vi "Log Error.vi"(8 "error in (no error)":errorcluster, 9 "error to log (no error)":errorcluster, 10 "Source Name":string, 11 "cRIO-CO2 in":refnum<class "cRIO-CO2.lvclass">) -> (0 "error out":errorcluster, 3 "cRIO-CO2 out":refnum<class "cRIO-CO2.lvclass">)   [LabVIEW 2015, in "cRIO-Carbondioxide.lvlib" / "cRIO-CO2.lvlib" / "cRIO-CO2.lvclass"]
uses:
  cRIO-CO2.lvclass
  <vilib>/Utility/error.llb/DialogType.ctl
  cRIO-CO2.lvclass/cRIO-CO2.ctl
  cRIO-CO2 Messages/Log Message Msg/Log Message Msg.lvclass/Log Message Msg.ctl
  <vilib>/ActorFramework/Message Enqueuer/Message Enqueuer.lvclass/Message Enqueuer.ctl
  <vilib>/ActorFramework/Message Enqueuer/Enqueue.vi
  <vilib>/ActorFramework/Message Priority Queue/Priority Enqueue.vi
  cRIO-CO2 Messages/Log Message Msg/Log Message Msg.lvclass
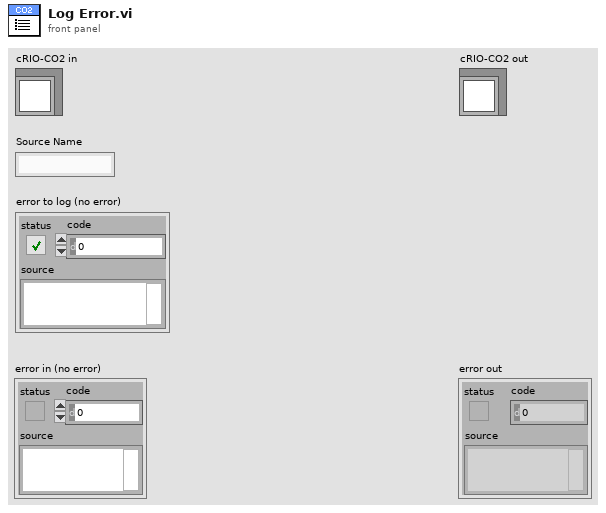
[diagram p1: front panel]
types:
  T1 = typedef "DialogType.ctl" = u16
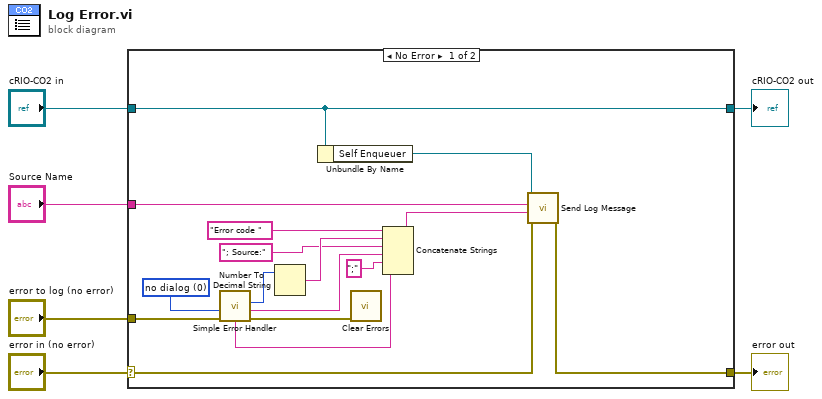
[diagram p0: block diagram]
diagram:
  n1 = case shown="No Error" "error in (no error)" {
    selector: "error in (no error)" -> [w12 w24]
    tunnel: [w11 w24] -> w5
    tunnel: [w14 w23] -> w3
    tunnel: "cRIO-CO2 in" -> [w14 w23]
    tunnel: "Source Name" -> [w10 _]
    tunnel: "error to log (no error)" -> [w21 _]
    frame No Error {
      w20 = T1 0 items=["no dialog", "OK message", "continue or stop message", "OK message + warnings", "continue/stop + warnings"] ("type of dialog (OK msg:1)")
      n2 = call <vilib>:"Simple Error Handler.vi"("type of dialog (OK msg:1)"=w20, "error in (no error)"=w21) -> ("code out"=w19:i32, "source out"=w8:string, "error out"=w7:errorcluster, "message"=w15:string)  [unwired: 3 in, 1 out]
      n3 = Number To Decimal String(number=w19) -> (decimal integer string=w18:string)  [unwired: 1 in]
      n4 = Unbundle By Name(w14) -> ("Self Enqueuer"=w13:refnum<class "Message Enqueuer.lvclass">)
      n5 = call <vilib>:"Clear Errors.vi"("error in (no error)"=w7) -> ()  [unwired: 5 in, 2 out]
      n6 = Concatenate Strings("Error code " ("string"), w18, "; Source:" ("string"), w8, ";" ("string"), w15) -> (w9:string)
      n7 = call "Send Log Message.vi"("error in (no error)"=w12, "String"=w9, "Source Name"=w10, "Message Enqueuer"=w13) -> ("error out"=w11:errorcluster)  [unwired: 6 in, 1 out]
    }
    frame Error {
    }
  }
  "error out" <- w5
  "cRIO-CO2 out" <- w3
